vi "Check Disabled.vi"(8 "error in (no error)":errorcluster, 10 "Array":T1(array[cluster]), 11 "LoggingControl in":refnum<class "LoggingControl.lvclass">) -> (0 "error out":errorcluster, 2 "All Logging":bool, 3 "LoggingControl out":refnum<class "LoggingControl.lvclass">)   [LabVIEW 2020, in "VolatusGUIElements.lvlib" / "LoggingControl.lvclass"]
uses:
  LoggingControl.lvclass
  LoggingControl.lvclass/LoggingControl.ctl
  VolatusData/Logging State.ctl
  VolatusData/VolatusData.lvlib
  VolatusGUI/GUI Element/GUI Element.lvclass
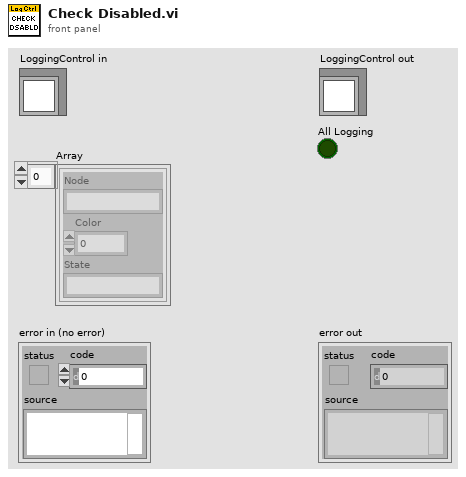
[diagram p1: front panel]
types:
  T1 = cluster{"Node":string, "Color":u32, "State":string}[]
  T2 = typedef "VolatusData.lvlib/Logging State.ctl" = enum16{"Idle", "Starting", "Logging", "Stopping"}
  T3 = enum8{"Enabled", "Disabled", "Disabled and Grayed Out"}
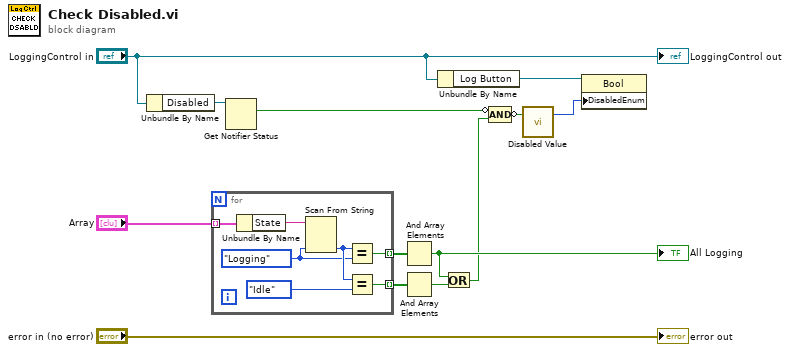
[diagram p0: block diagram]
diagram:
  n1 = Unbundle By Name("LoggingControl in") -> ("Disabled"=w5:refnum<notifier>)
  n2 = for {
    tunnel: "Array" -> [w20] mode=indexing
    tunnel: [w15] -> w11 mode=indexing
    tunnel: [w14] -> w10 mode=indexing
    w16 = Logging_State."Logging" ("Logging State")
    n3 = Unbundle By Name(w20) -> ("State"=w19:string)
    n4 = Scan From String(input string=w19, default 1=w16) -> (output 1=w17:T2)  [unwired: 3 in, 3 out]
    n5 = Equal?(x=w17, y=w16) -> (x = y?=w15:bool)
    n6 = Equal?(x=w17, y=Logging_State."Idle") -> (x = y?=w14:bool)
  }
  n7 = Get Notifier Status(notifier=w5) -> (current notification=w4:bool)  [unwired: 1 in, 4 out]
  n8 = And Array Elements(Boolean array=w11) -> (logical AND=w9:bool)
  "All Logging" <- w9
  n9 = And Array Elements(Boolean array=w10) -> (logical AND=w8:bool)
  n10 = Unbundle By Name("LoggingControl in") -> ("Log Button"=w7:refnum<vi>)
  n11 = Or(x=w9, y=w8) -> (x .or. y?=w3:bool)
  n12 = Compound Arithmetic op=AND(invert w4, w3) -> (invert w2:bool)
  n13 = call "Disabled Value.vi"("Disabled"=w2) -> ("Disabled Value"=w1:T3)  [unwired: 6 in]
  n14 = property class="Bool"(reference=w7, "DisabledEnum"=w1) -> ()  [unwired: 1 in, 2 out]
  "error out" <- "error in (no error)"
  "LoggingControl out" <- "LoggingControl in"
